vi "PH_Timing.Action link PUs.vi"(0 "i ref in":refnum<vi>, 2 "PU index":T1, 5 "error in (no error)":errorcluster) -> (14 "i ref out":refnum<vi>, 19 "error out":errorcluster)   [LabVIEW 2014, in "PH_Timing.lvlib"]
doc: "Within this VI the action of the related event case is done: gate generators in total or channls are en- or disabled depending on the state of the related power unit."
uses:
  PH_Timing.lvlib
  PH_Basics/PH_PP_Common/PH_PP_Common.PUs.ctl
  CS_DigitalIO/BNC555/BNC555.lvlib
  PH_Basics/PH_PP_Common/PH_PP_Common.lvlib
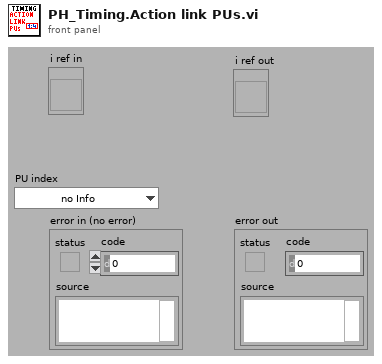
[diagram p1: front panel]
types:
  T1 = typedef "PH_PP_Common.lvlib/PH_PP_Common.PUs.ctl" = enum16{"no Info", "PA-19mm-1", "PA-19mm-2", "PA-45mm-PILC", "PA-45mm-MAIN", "MA-PU-1", "MA-PU-2", "MA-PU-3", "MA-PU-4", "MA-PU-5", "MA-PU-6", "MA-FR", "MA-PILC", "PA-45mm-DP"}
  T2 = typedef "PH_Timing.lvlib/PH_Timing.i attribute.ctl" = cluster{"Sequencer":cluster{"linked?":bool, "Proc State":string, "Ref State":refnum<vi>}, "Gate Generator":cluster{"GD":cluster{"Device Status":T3, "linked?":bool}, "Settings":T4, "GUI Ref":refnum<vi>}, "Interlock Bypass":cluster{"Instancename":string, "Switch linked?":bool, "Device Status":T3, "Ref Status":refnum<vi>}, "Roughtuner":cluster{"Settings":T5, "GUI Ref":refnum<vi>, "GD":cluster{"Device Status":T3, "linked?":bool}}, "0,5Hz Gater":cluster{"Settings":T6, "GUI Ref":refnum<vi>, "GD":cluster{"Device Status":T3, "linked?":bool}}, "Slow Trigger":cluster{"Settings":T7, "GUI Ref":refnum<vi>, "Service ID Delay":i32, "Service ID Ext Trig":i32, "Wanted Settings":T7}, "Timing Mode":cluster{"Mode":T8, "GUI Ref":refnum<vi>, "Service ID T2":i32, "Service ID Mode":i32, "Wanted Mode":T8}, "ns Generator":cluster{"Settings":T9, "ns Generator Settings":refnum<vi>, "GD":cluster{"Device Status":T3, "linked?":bool}}, "Phase FEs":cluster{"Settings":T12, "GUI Ref":refnum<vi>, "Service ID Phase":i32, "Wanted Settings":T12}, "GD GUI Refs":refnum<vi>[], "Heads":T13[], "GUI Ref Delete":refnum<vi>}
  T3 = typedef "PH_StatusHandler.lvlib/PH_StatusHandler.Status.ctl" = i16
  T4 = typedef "PH_Timing.lvlib/PH_Timing.GateGen.ctl" = cluster{"Instance":string, "Channel Gate":i32, "Channel T2":i32, "Width Gate":dbl, "Width T2":dbl, "Delay Gate":dbl, "Delay T2":dbl, "Gate activ":bool, "T2 activ":bool, "System Mode":enum16{"Normal", "Single", "Burst", "Duty Cycle"}}
  T5 = typedef "PH_Timing.lvlib/PH_Timing.Roughtuner.ctl" = cluster{"Instance":string, "Phase PHELIX / UNILAC":cluster{"Channel":u16, "relative to":u16, "Delay [ms]":dbl}, "Pulse Length":cluster{"Channel":u16, "relative to":u16, "Delay [ms]":dbl}, "Trigger":cluster{"externally?":bool, "Rate [Hz]":dbl}}
  T6 = typedef "PH_Timing.lvlib/PH_Timing.0.5HzGater.ctl" = cluster{"Instance":string, "Channel ns FE Delay":i32, "Channel 0.5Hz":i32, "Width ns FE Delay":dbl, "Width 0.5Hz":dbl, "Delay ns FE Delay":dbl, "Delay 0.5Hz":dbl, "ns FE Delay active":bool, "0.5Hz activ":bool, "ns FE Delay inverted":bool, "0.5Hz inverted":bool}
  T7 = typedef "PH_Timing.lvlib/PH_Timing.Slow Trigger Settings.ctl" = cluster{"Delay":dbl, "externally triggered?":bool}
  T8 = typedef "PH_Timing.lvlib/PH_Timing.Timing Mode.ctl" = cluster{"T2":i16, "Modeselector":enum32{"10 Hz", "0.5 Hz", "Shot"}}
  T9 = typedef "PH_Timing.lvlib/PH_Timing.ns Generator.ctl" = cluster{"Instance":string, "Phase fs / ns FE":cluster{"Channel":T10, "Settings":T11}}
  T10 = typedef "Stanford Research DG645 - Driver.lvlib/Channel.ctl" = i32
  T11 = typedef "PH_SRDG645.lvlib/PH_SRDG645.Channel Settings.ctl" = cluster{"Delay [s]":dbl, "relative to":i32}
  T12 = typedef "PH_Timing.lvlib/PH_Timing.Phase FEs.ctl" = cluster{"Phase":dbl}
  T13 = typedef "PH_Timing.lvlib/PH_Timing.PU Data.ctl" = cluster{"linked?":bool, "Data":T14, "GD":cluster{"Device Status":T3, "linked?":bool}, "GUI Ref":refnum<vi>, "PU":T1}
  T14 = typedef "PH_Timing.lvlib/PH_Timing.PU Info.ctl" = cluster{"Act CH?":bool, "GD":string, "CH":i32, "Delay":dbl, "active":bool, "in Use?":bool}
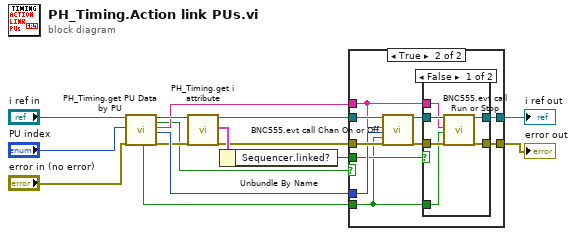
[diagram p0: block diagram]
diagram:
  n1 = call "PH_Timing.get PU Data by PU.vi"("VI in"="i ref in", "PU"="PU index", "error in (no error)"="error in (no error)") -> ("Activate Channel?"=w7:bool, "VI out"=w3:refnum<vi>, "GD linked?"=w1:bool, "GD Name"=w2:string, "CH"=w8:i32, "error out"=w5:errorcluster)  [unwired: 9 in, 2 out]
  n2 = call "PH_Timing.get i attribute.vi"("i ref in"=w3, "error in (no error)"=w5) -> ("i ref out"=w15:refnum<vi>, "i attribute"=w13:T2, "error out"=w10:errorcluster)  [unwired: 15 in]
  n3 = Unbundle By Name(w13) -> ("Sequencer.linked?"=w12:bool)
  n4 = case shown="True" w1 {
    tunnel: w15 -> [w17 w27]
    tunnel: [w17 w26] -> w14
    tunnel: w10 -> [w16 w25]
    tunnel: w8 -> [_ w24]
    tunnel: w12 -> [_ w23]
    tunnel: [w16 w21] -> w11
    tunnel: w2 -> [_ w22]
    tunnel: w7 -> [_ w20]
    frame False {
    }
    frame True {
      n5 = call "BNC555.evt call Chan On or Off.vi"("i ref in"=w27, "Generator Instance"=w22, "Channel"=w24, "State"=w20, "error in (no error)"=w25) -> ("i ref out"=w19:refnum<vi>, "error out"=w18:errorcluster)  [unwired: 13 in]
      n6 = case shown="False" w23 {
        tunnel: w19 -> [w33 w34]
        tunnel: w18 -> [w32 w35]
        tunnel: w22 -> [w31 _]
        tunnel: [w30 w34] -> w26
        tunnel: [w28 w35] -> w21
        tunnel: w20 -> [w29 _]
        frame False {
          n7 = call "BNC555.evt call Run or Stop.vi"("i ref in"=w33, "Generator Instance"=w31, "Start\\Stop"=w29, "error in (no error)"=w32) -> ("i ref out"=w30:refnum<vi>, "error out"=w28:errorcluster)  [unwired: 14 in]
        }
        frame True {
        }
      }
    }
  }
  "error out" <- w11
  "i ref out" <- w14
